vi "GetTemperatureData.vi"(8 "error in":errorcluster, 9 "Length":i32=250, 11 "ON":bool) -> (0 "error out":errorcluster, 2 "Temperature":dbl)   [LabVIEW 2012]
uses:
  GlobalVariables/HardwarePresent.vi
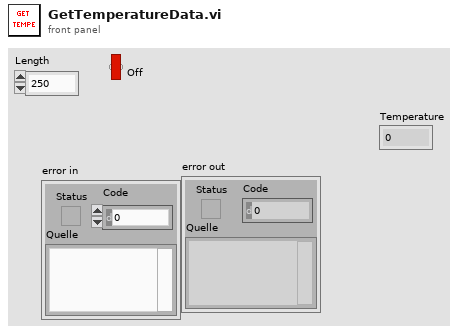
[diagram p1: front panel]
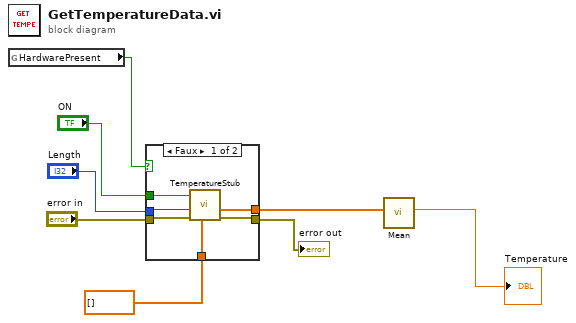
[diagram p0: block diagram]
diagram:
  n1 = global read "HardwarePresent.vi" "HardwarePresent"() -> (w5:bool)
  n2 = case shown="Faux" w5 {
    tunnel: "error in" -> [w13 w16]
    tunnel: [w14 w16] -> w4
    tunnel: "Length" -> [w12 _]
    tunnel: "ON" -> [w11 _]
    tunnel: [w10 w15] -> w2
    tunnel: dbl[] [] ("FittedPolynomCoeffsServices") -> [w9 w15]
    frame False {
      n3 = call "TemperatureStub.vi"("TemperatureIn"=w9, "error in"=w13, "Length"=w12, "ON"=w11) -> ("error out"=w14:errorcluster, "TemperatureOut"=w10:dbl[])  [unwired: 6 in]
    }
    frame True {
    }
  }
  "error out" <- w4
  n4 = call "Mean.vi"("Array"=w2) -> ("Mean"=→"Temperature":dbl)  [unwired: 10 in]
